vi "WFGConfigureFMMODSingleCh.vi"(0 "object in":refnum<class "AD2_WFG_SDK.lvclass">, 2 "Ch":T1={"idxChannel"=0, "Settings out of range"=FALSE, "Carrier"={"Frequency (Hz)"=1000.0, "Amplitude (V)"=1.0, "Offset(V)"=0.0, "Symmetry(%) "=50.0, "Phase(Deg)"=0.0, "Function"=1, "Enable"=FALSE}, "Trigger"={"secRun(0=Cont)"=0.0, "secWait"=0.0, "cRepeat(0=inf)"=0, "Repeat Trigger"=FALSE, "TrigrSrc"=enum."trigrsrcNone"}, "FM Mod"={"Frequency (Hz)"=1000.0, "Amplitude (%)"=1.0, "Offset(V)"=0.0, "Symmetry(%) "=50.0, "Phase(Deg)"=0.0, "Function 2"=1, "Enable"=FALSE}} {"FM Mod"."Function 2" items=["DC"=0, "Sine"=1, "Square"=2, "Triangle"=3, "RampUp"=4, "RampDown"=5, "Noise"=6, "Pulse"=7, "Custom"=30]; "Carrier"."Function" items=["DC"=0, "Sine"=1, "Square"=2, "Triangle"=3, "RampUp"=4, "RampDown"=5, "Noise"=6, "Pulse"=7, "Custom"=30]}, 5 "error in (no error)":errorcluster) -> (14 "object out":refnum<class "AD2_WFG_SDK.lvclass">, 19 "error out":errorcluster)   [LabVIEW 2021, in "AD2_WFG_SDK.lvclass"]
uses:
  AD2_WFG_SDK.lvclass
  WFGCh.ctl
  AD2TriggerSources.ctl
  Olasdwf/Olasdwf.lvlib
  AD2_SDK_class/AD2_SDK.lvclass
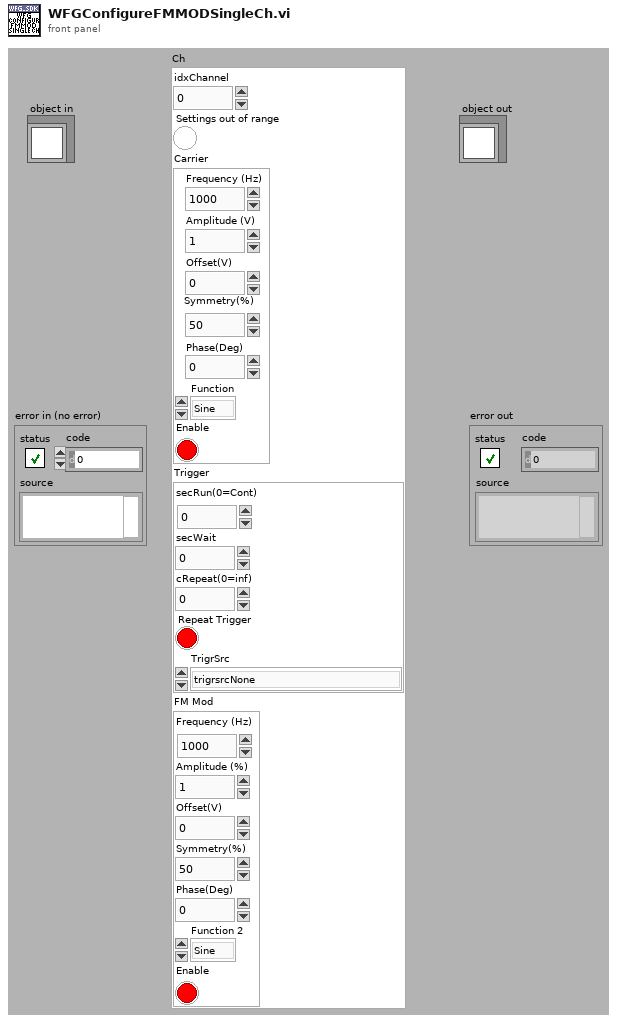
[diagram p1: front panel]
types:
  T1 = typedef "AD2_WFG_SDK.lvclass/WFGCh.ctl" = cluster{"idxChannel":i32, "Settings out of range":bool, "Carrier":cluster{"Frequency (Hz)":dbl, "Amplitude (V)":dbl, "Offset(V)":dbl, "Symmetry(%) ":dbl, "Phase(Deg)":dbl, "Function":u16, "Enable":bool}, "Trigger":cluster{"secRun(0=Cont)":dbl, "secWait":dbl, "cRepeat(0=inf)":i32, "Repeat Trigger":bool, "TrigrSrc":T2}, "FM Mod":cluster{"Frequency (Hz)":dbl, "Amplitude (%)":dbl, "Offset(V)":dbl, "Symmetry(%) ":dbl, "Phase(Deg)":dbl, "Function 2":u16, "Enable":bool}}
  T2 = typedef "AD2_SDK.lvclass/AD2TriggerSources.ctl" = enum8{"trigrsrcNone", "trigsrcPC", "trigsrcDetectorAnalogIn", "trigsrcDetectorDigitalIn", "trigsrcAnalogIn", "trigsrcDigitalIn", "trigsrcDigitalOut", "trigsrcAnalogOut1", "trigsrcAnalogOut2", "trigsrcAnalogOut3", "trigsrcAnalogOut4", "trigsrcExternal1", "trigsrcExternal2", "trigsrcExternal3", "trigsrcExternal4", ""}
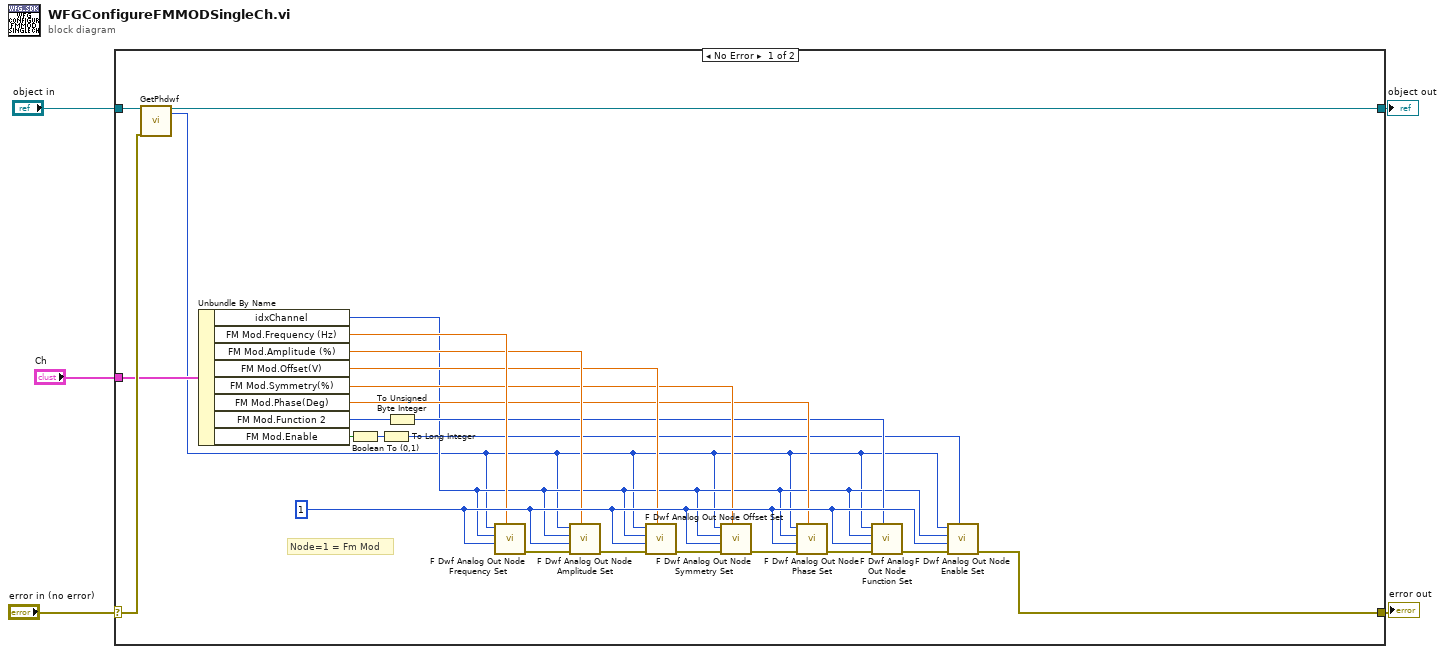
[diagram p0: block diagram]
diagram:
  n1 = case shown="No Error" "error in (no error)" {
    selector: "error in (no error)" -> [w24 w31]
    tunnel: [w8 w31] -> w4
    tunnel: [w26 w30] -> w2
    tunnel: "object in" -> [w25 w30]
    tunnel: "Ch" -> [w23 _]
    frame No Error {
      w16 = 1 ("node")
      # "Node=1 = Fm Mod"
      n2 = call-dynamic "GetPhdwf.vi"("object in"=w25, "error in (no error)"=w24) -> ("object out"=w26:refnum<class "AD2_WFG_SDK.lvclass">, "phdwf"=w6:i32)  [unwired: 15 in, 1 out]
      n3 = Unbundle By Name(w23) -> ("idxChannel"=w7:i32, "FM Mod.Frequency (Hz)"=w15:dbl, "FM Mod.Amplitude (%)"=w14:dbl, "FM Mod.Offset(V)"=w13:dbl, "FM Mod.Symmetry(%)"=w12:dbl, "FM Mod.Phase(Deg)"=w11:dbl, "FM Mod.Function 2"=w28:u16, "FM Mod.Enable"=w27:bool)
      n4 = Boolean To (0,1)(Boolean=w27) -> (0, 1=w29:i16)
      n5 = To Long Integer(number=w29) -> (32bit integer=w9:i32)
      n6 = To Unsigned Byte Integer(number=w28) -> (unsigned 8bit integer=w10:u8)
      n7 = call "F Dwf Analog Out Node Frequency Set.vi"("hzFrequency"=w15, "node"=w16, "idxChannel"=w7, "hdwf"=w6) -> ("error out"=w18:errorcluster)  [unwired: 6 in, 1 out]
      n8 = call "F Dwf Analog Out Node Amplitude Set.vi"("vAmplitude"=w14, "error in (no error)"=w18, "node"=w16, "idxChannel"=w7, "hdwf"=w6) -> ("error out"=w19:errorcluster)  [unwired: 5 in, 1 out]
      n9 = call "F Dwf Analog Out Node Offset Set.vi"("vOffset"=w13, "error in (no error)"=w19, "node"=w16, "idxChannel"=w7, "hdwf"=w6) -> ("error out"=w20:errorcluster)  [unwired: 5 in, 1 out]
      n10 = call "F Dwf Analog Out Node Symmetry Set.vi"("percentageSymmetry"=w12, "error in (no error)"=w20, "node"=w16, "idxChannel"=w7, "hdwf"=w6) -> ("error out"=w21:errorcluster)  [unwired: 5 in, 1 out]
      n11 = call "F Dwf Analog Out Node Phase Set.vi"("degreePhase"=w11, "error in (no error)"=w21, "node"=w16, "idxChannel"=w7, "hdwf"=w6) -> ("error out"=w22:errorcluster)  [unwired: 5 in, 1 out]
      n12 = call "F Dwf Analog Out Node Function Set.vi"("func"=w10, "error in (no error)"=w22, "node"=w16, "idxChannel"=w7, "hdwf"=w6) -> ("error out"=w17:errorcluster)  [unwired: 5 in, 1 out]
      n13 = call "F Dwf Analog Out Node Enable Set.vi"("fEnable"=w9, "error in (no error)"=w17, "node"=w16, "idxChannel"=w7, "hdwf"=w6) -> ("error out"=w8:errorcluster)  [unwired: 5 in, 1 out]
    }
    frame Error {
    }
  }
  "error out" <- w4
  "object out" <- w2
